vi "Uninstall Routine.vi"   [LabVIEW 2013]
uses:
  <vilib>/Utility/sysdir.llb/System Directory Type.ctl
panel:
  # "Removing extracted dependencies.\n\n\nPlease wait..."
types:
  T1 = typedef "System Directory Type.ctl" = i32
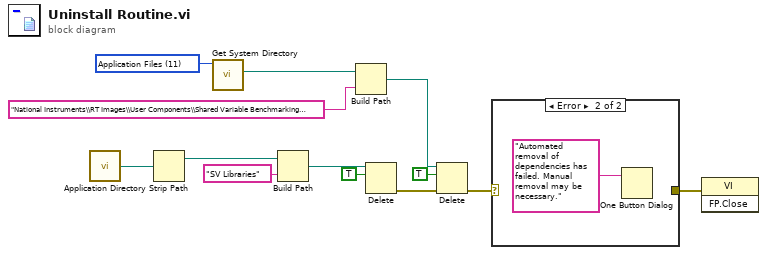
[diagram p0: block diagram]
diagram:
  w13 = T1 11 items=["User Home"=0, "User Desktop"=1, "User Documents"=2, "User Application Data"=3, "User Preferences"=4, "User Temporary"=5, "Public Documents"=6, "Public Application Data"=7, "Public Preferences"=8, "Public Cache"=13, "System Core Libraries"=9, "System Installed Libraries"=10, "Application Files"=11, "Boot Volume Root"=12] ("system directory type")
  n1 = call <vilib>:"Application Directory.vi"() -> ("Application Directory"=w10:path)
  n2 = Strip Path(path=w10) -> (stripped path=w9:path)  [unwired: 1 out]
  n3 = call <vilib>:"Get System Directory.vi"("system directory type"=w13) -> ("system directory"=w12:path)  [unwired: 10 in]
  n4 = Build Path(base path=w9, name or relative path="SV Libraries") -> (appended path=w7:path)
  n5 = Build Path(base path=w12, name or relative path="National Instruments\\RT Images\\User Components\\Shared Variable Benchmarking Utility") -> (appended path=w5:path)
  n6 = Delete(path (use dialog)=w7, entire hierarchy (F)=TRUE) -> (error out=w4:errorcluster)  [unwired: 3 in, 2 out]
  n7 = Delete(path (use dialog)=w5, entire hierarchy (F)=TRUE, error in=w4) -> (error out=w1:errorcluster)  [unwired: 2 in, 2 out]
  n8 = case shown="Error" w1 {
    selector: w1 -> [w14 _]
    tunnel: [w14 _] -> w2
    frame No Error {
    }
    frame Error {
      n9 = One Button Dialog(message="Automated removal of dependencies has failed. Manual removal may be necessary.") -> ()  [unwired: 1 in, 1 out]
    }
  }
  n10 = invoke class="VI" method="FP.Close"(error in=w2) -> ()  [unwired: 2 in, 3 out]
